vi "Tare IMU.vi"(8 "error in":errorcluster {"code" format="%.0x"}, 11 "Session In":refnum<visa-resource-name>) -> (0 "error out":errorcluster {"code" format="%.0x"}, 3 "Session Out":refnum<visa-resource-name>)   [LabVIEW 2012, in "YOST 3 Space.lvlib"]
uses:
  YOST 3 Space.lvlib
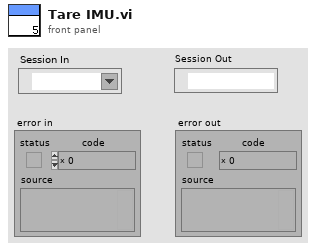
[diagram p1: front panel]
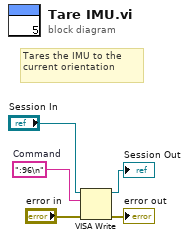
[diagram p0: block diagram]
diagram:
  w1 = ":96\n"  # Command
  # "Tares the IMU to the current orientation"
  n1 = VISA Write(VISA resource name="Session In", write buffer=w1, error in (no error)="error in") -> (VISA resource name out=→"Session Out":refnum<visa-resource-name>, error out=→"error out":errorcluster)  [unwired: 1 out]
